vi "scaler64_digital.vi"(7 "PresetValues_Scaler":u32[](array[numeric])=[0, 0, 0, 0, 0, 0, 0, 0, 0, 0, 0, 0, 0, 0, 0, 0, 0, 0, 0, 0, 0, 0, 0, 0, 0, 0, 0, 0, 0, 0, 0, 0, 0, 0, 0, 0, 0, 0, 0, 0, 0, 0, 0, 0, 0, 0, 0, 0, 0, 0, 0, 0, 0, 0, 0, 0, 0, 0, 0, 0, 0, 0, 0, 0], 8 "Pulse_Scaler":bool[](array[boolean])=[FALSE, FALSE, FALSE, FALSE, FALSE, FALSE, FALSE, FALSE, FALSE, FALSE, FALSE, FALSE, FALSE, FALSE, FALSE, FALSE, FALSE, FALSE, FALSE, FALSE, FALSE, FALSE, FALSE, FALSE, FALSE, FALSE, FALSE, FALSE, FALSE, FALSE, FALSE, FALSE, FALSE, FALSE, FALSE, FALSE, FALSE, FALSE, FALSE, FALSE, FALSE, FALSE, FALSE, FALSE, FALSE, FALSE, FALSE, FALSE, FALSE, FALSE, FALSE, FALSE, FALSE, FALSE, FALSE, FALSE, FALSE, FALSE, FALSE, FALSE, FALSE, FALSE, FALSE, FALSE], 9 "Gate_Scaler":bool[](array[boolean])=[FALSE, FALSE, FALSE, FALSE, FALSE, FALSE, FALSE, FALSE, FALSE, FALSE, FALSE, FALSE, FALSE, FALSE, FALSE, FALSE, FALSE, FALSE, FALSE, FALSE, FALSE, FALSE, FALSE, FALSE, FALSE, FALSE, FALSE, FALSE, FALSE, FALSE, FALSE, FALSE, FALSE, FALSE, FALSE, FALSE, FALSE, FALSE, FALSE, FALSE, FALSE, FALSE, FALSE, FALSE, FALSE, FALSE, FALSE, FALSE, FALSE, FALSE, FALSE, FALSE, FALSE, FALSE, FALSE, FALSE, FALSE, FALSE, FALSE, FALSE, FALSE, FALSE, FALSE, FALSE], 10 "OneShot_Scaler":bool, 11 "Enable_Scaler":bool) -> (0 "Counter_Scaler":u32[](array[numeric]), 3 "Done_Scaler":bool)   [LabVIEW 2017, in "scaler.lvlib"]
uses:
  scaler.lvlib
panel:
  # "This is a 64 channel digital scaler. It follows to the word the definition of the scaler in the anl website\nhttps://epics.anl.gov/bcda/synApps/std/scalerRecord.html"
  # "Optimization tip:\nMake all the arrays the same size as the number\nof channels you need implemented. Setting\nthe number of channels uses up to 45% of the \nresources. Setting to 2 uses only 23%."
  # "Input and output description\n - Gate_Scaler[64] : corresponds to 64 counters S1-S64\n - Pulse_Scaler[63] : corresponds to 63 counters S2-S64\n - PresetValues_Scaler[64]: corresponds to 64 counters S1-S64\n - OneShot_Scaler: Oneshot / autocount is also implemented \n                                 in hardware. When necessary, can be used.\n                                 When not necessary (implmented in software)\n                                 this port can be fixed to 1.\n - Counter_Scaler[64]: 64 counter readings.\n - Done_Scaler : Done signal as per Scaler specifications\n - Enable_Scaler: Set to one when CNT is set to 1."
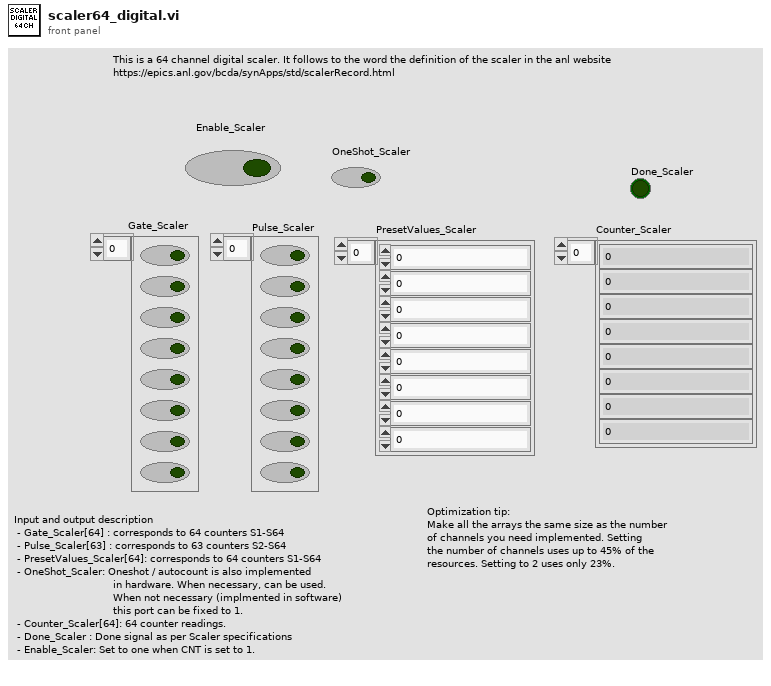
[diagram p1: front panel]
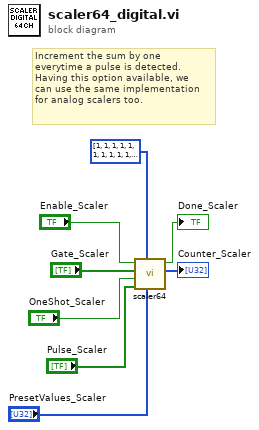
[diagram p0: block diagram]
diagram:
  # "Increment the sum by one\neverytime a pulse is detected.\nHaving this option available, we \ncan use the same implementation\nfor analog scalers too."
  n1 = call "scaler64.vi"("PresetValues_Scaler"="PresetValues_Scaler", "AnalogInputs_Scaler"=u32[] [1, 1, 1, 1, 1, 1, 1, 1, 1, 1, 1, 1, 1, 1, 1, 1, 1, 1, 1, 1, 1, 1, 1, 1, 1, 1, 1, 1, 1, 1, 1, 1, 1, 1, 1, 1, 1, 1, 1, 1, 1, 1, 1, 1, 1, 1, 1, 1, 1, 1, 1, 1, 1, 1, 1, 1, 1, 1, 1, 1, 1, 1, 1, 1], "Pulse_Scaler"="Pulse_Scaler", "OneShot_Scaler"="OneShot_Scaler", "Gate_Scaler"="Gate_Scaler", "Enable_Scaler"="Enable_Scaler") -> ("Counter_Scaler"=→"Counter_Scaler":u32[], "Done_Scaler"=→"Done_Scaler":bool)  [unwired: 4 in]
